vi "ReadForceSensor.vi"() -> ()   [LabVIEW 2011]
uses:
  sensor_list.ctl
  statesReadForceSensor.ctl
  QueueCtl.ctl
  <vilib>/DAQmx/read.llb/DAQmx Read (Analog DBL 1Chan 1Samp).vi
  <vilib>/DAQmx/create/channels.llb/DAQmx Create Channel (AI-Voltage-Basic).vi
  <vilib>/DAQmx/miscellaneous.llb/DAQmx Fill In Error Info.vi
  <vilib>/Utility/file.llb/Write To Spreadsheet File (DBL).vi
panel:
  in  "channels":tag
  in  "Previous":bool
  in  "Bumper":T1(ring)
  in  "Number of observations":i32=5
  in  "weight sequence (g)":dbl[](array[numeric])=[0.0, 50.0, 100.0, 200.0, 426.6, 1000.0, 1870.0, 2820.0, 3700.0, 5559.0, 6559.0, 7419.0, 9239.0]
  in  "Apparatus wt (g)":dbl=183.5
  in  "Unit number":string
  in  "Sensor model":T2=enum."interlink-FSR"
  out "standard error":string
  out "standard output":string
  in  "play python":bool
  in  "Data (CSV) path":path
  out "display":string="Remove all weights,\npull up the rod-setup and \npress \"NEXT\""
  in  "Next Button":bool
  out "Value (mV)":dbl
  out "Place weight (g)":dbl
  out "error out":errorcluster
  # "FORCE SENSOR - DEAD WEIGHT TEST"
  # "Settings:"
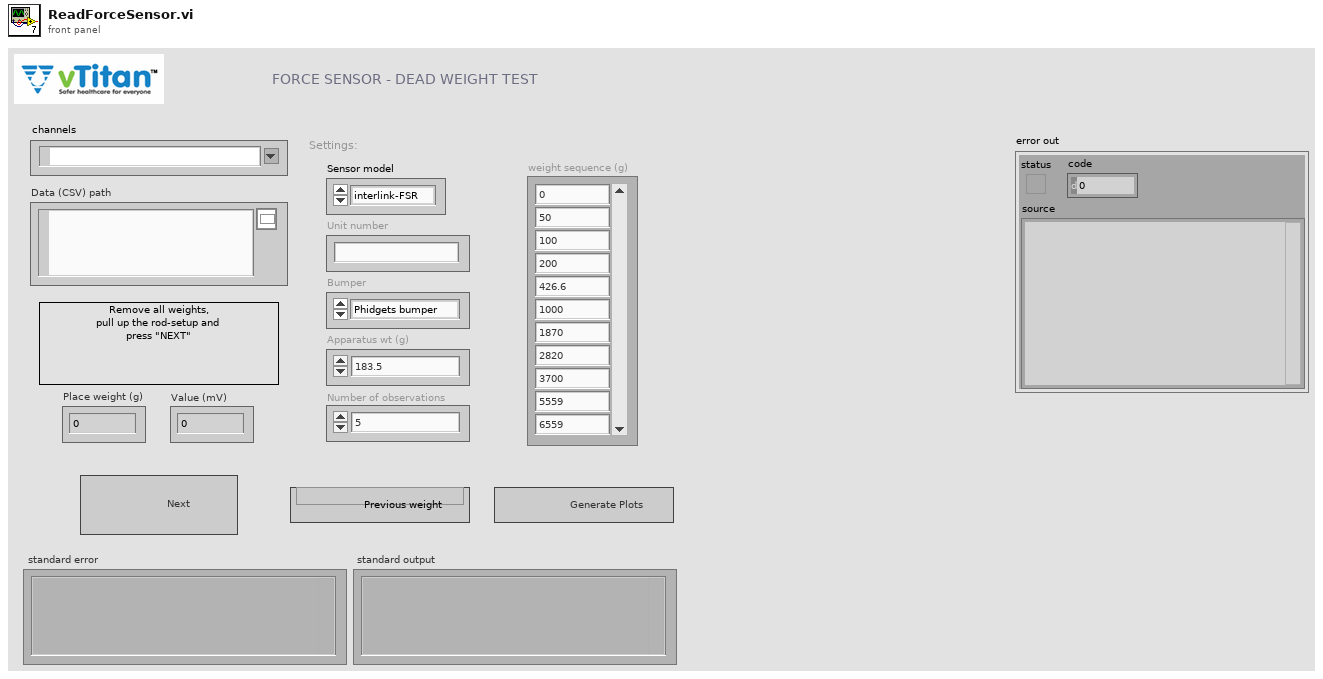
[diagram p1: front panel]
types:
  T1 = enum16{"Phidgets bumper", "Plastic bumper", "neoprene rubber"}
  T2 = typedef "sensor_list.ctl" = enum16{"ESS301", "FSG005WNPB", "FSG010WNPB", "FSG015WNPB", "FSS010WNGT", "FSS015WNGT", "A201", "interlink-FSR", "sensitronics-FSR", "NPI-12"}
  T3 = typedef "QueueCtl.ctl" = enum16{"Create", "Enqueue-N", "Dequeue - 1 ", "Enstack - N", "Flush", "Release"}
  T4 = cluster{"reading":dbl, "nul_offset":dbl, "device_ref":refnum<k21>, "weights":i32[], "data":dbl[][], "excel_path":path, "count":i32, "num_read":i32, "next":bool, "state_meas":enum16{"to_read_null", "to_read_value"}, "script_relpath":string}
  T5 = typedef "statesReadForceSensor.ctl" = enum16{"initialize", "poll", "find null offset", "measure value", "write to file", "remeasure weight", "display", "run python scripts", "exit"}
  T6 = enum16{"ESS301", "FSG005WNPB", "FSG010WNPB", "FSG015WNPB", "FSS010WNGT", "FSS015WNGT", "A201", "interlink-FSR", "sensitronics-FSR", "NPI-12"}
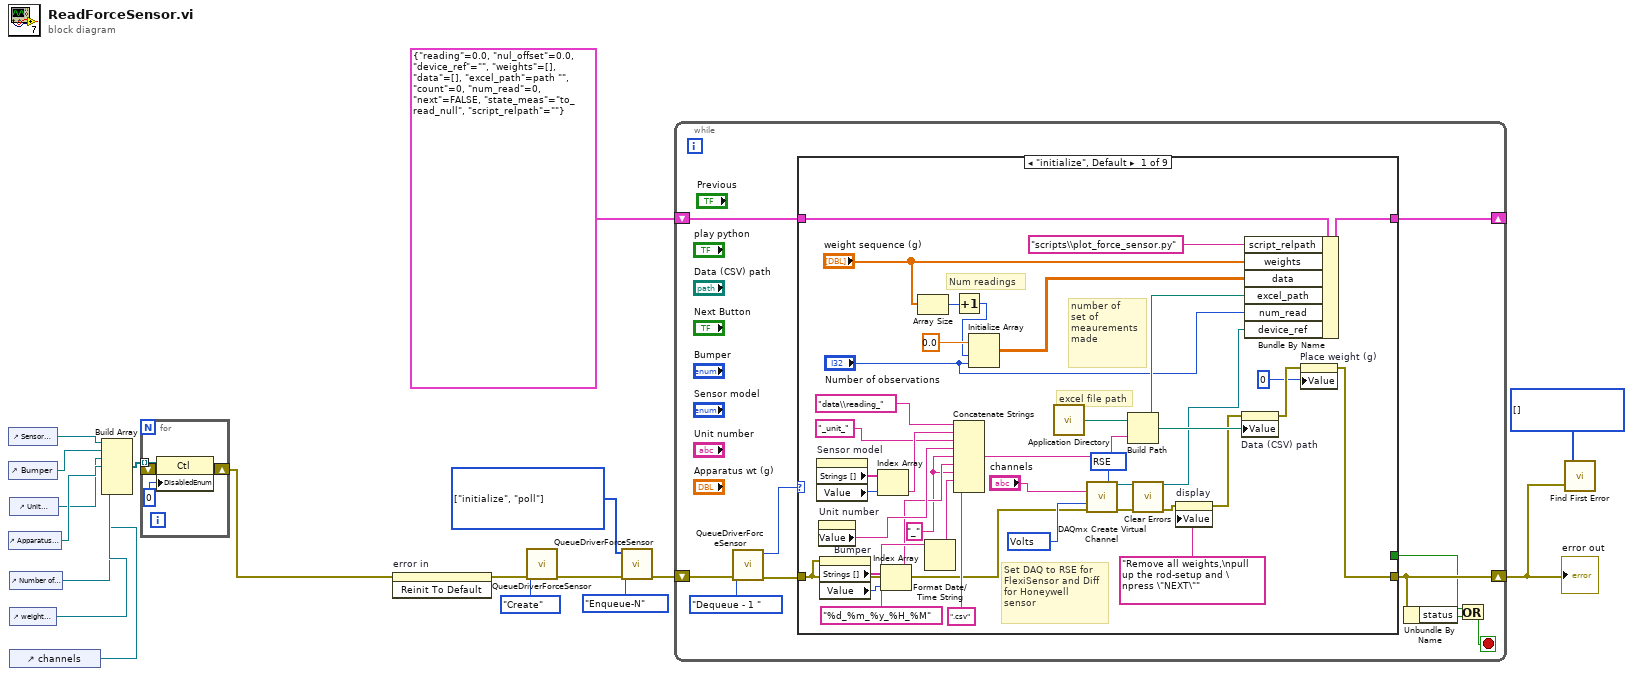
[diagram p0: block diagram]
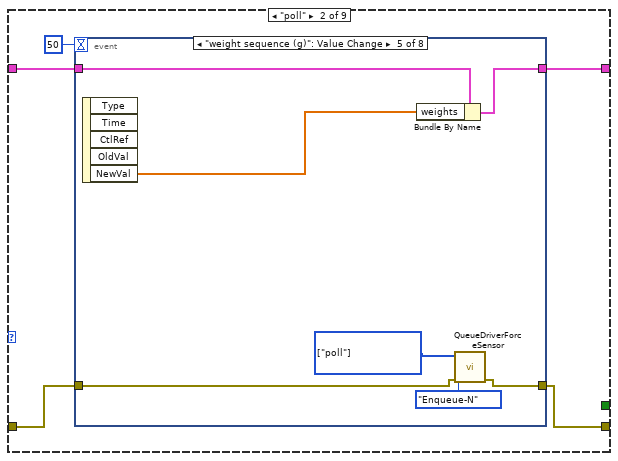
[diagram p2: hidden frame]
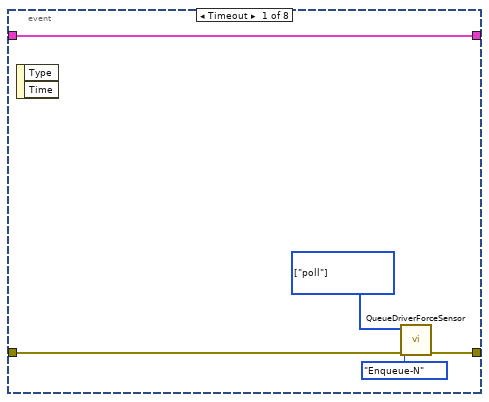
[diagram p3: hidden frame]
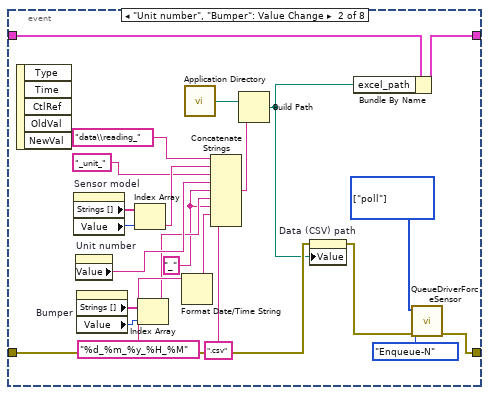
[diagram p4: hidden frame]
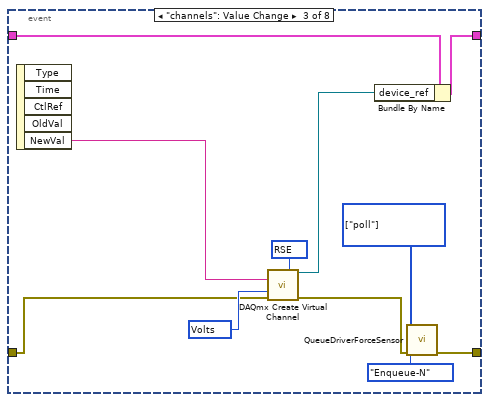
[diagram p5: hidden frame]
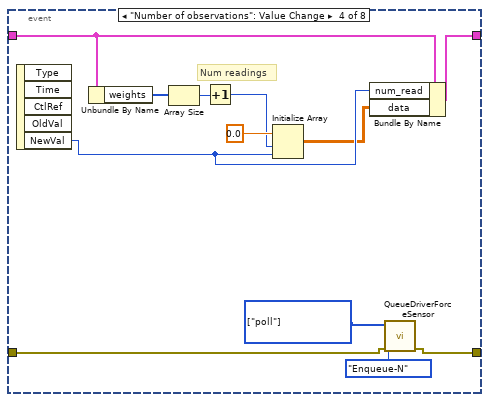
[diagram p6: hidden frame]
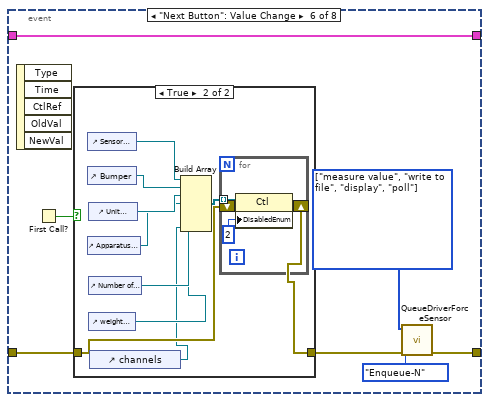
[diagram p7: hidden frame]
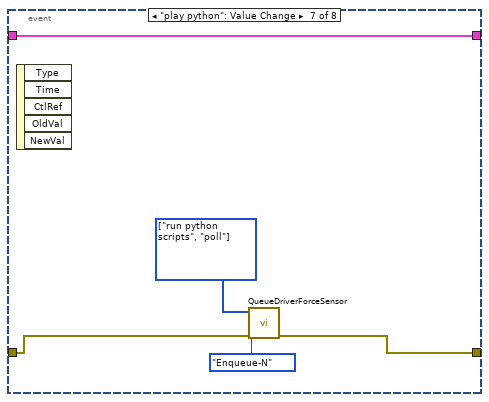
[diagram p9: hidden frame]
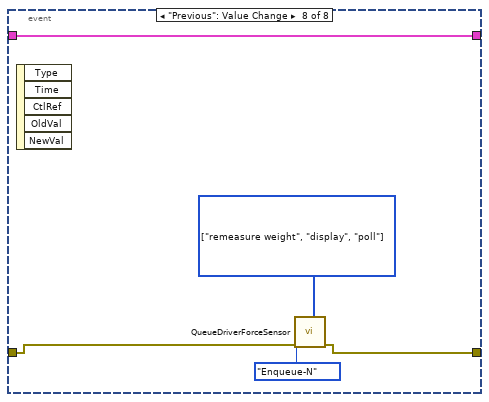
[diagram p10: hidden frame]
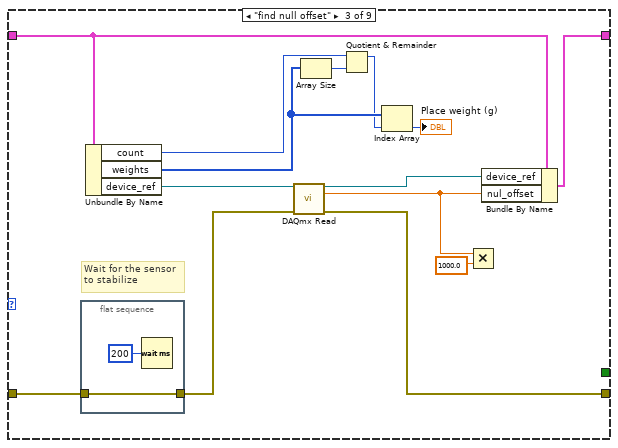
[diagram p11: hidden frame]
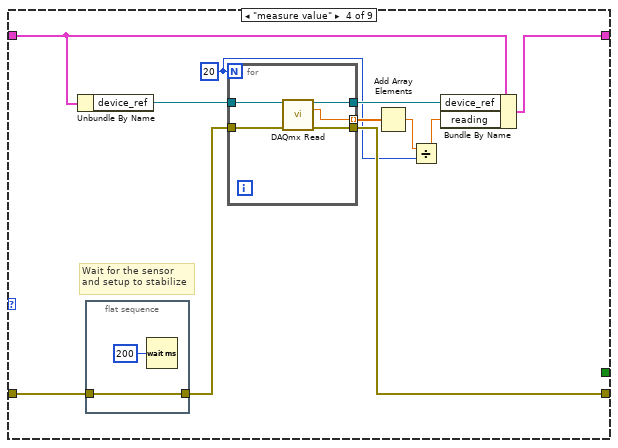
[diagram p12: hidden frame]
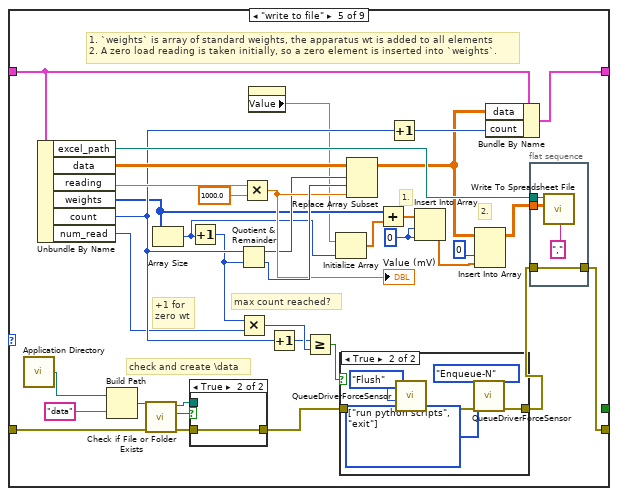
[diagram p13: hidden frame]
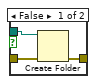
[diagram p15: hidden frame]
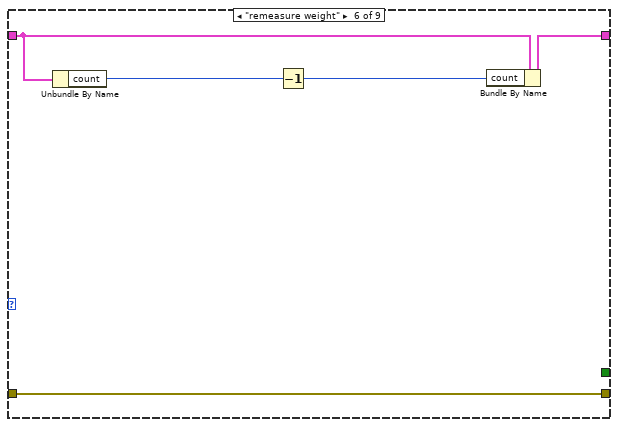
[diagram p16: hidden frame]
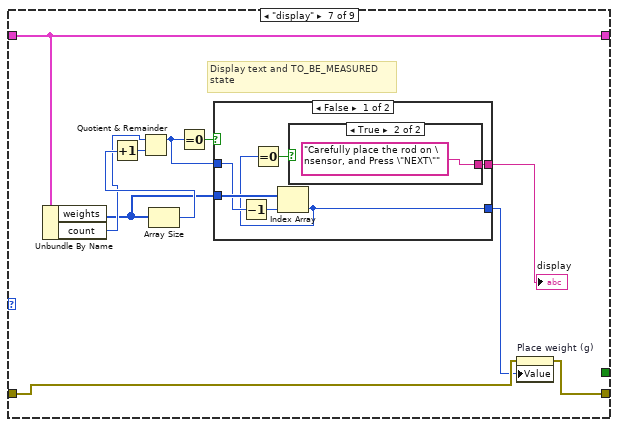
[diagram p17: hidden frame]
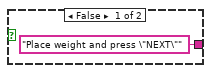
[diagram p18: hidden frame]
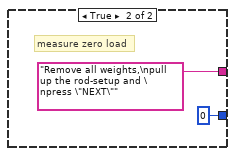
[diagram p19: hidden frame]
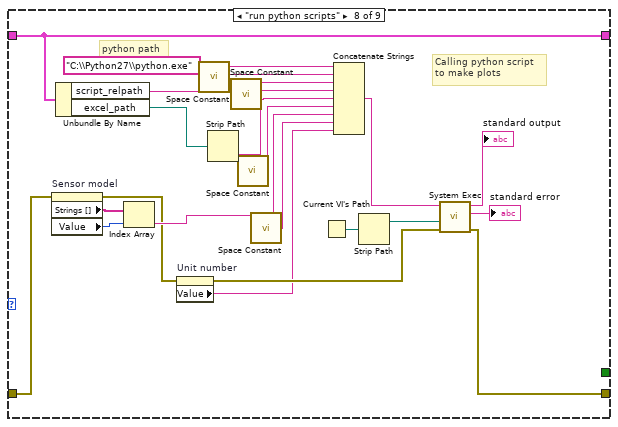
[diagram p20: hidden frame]
diagram:
  w11 = T5[] [enum."initialize", enum."poll"] items=["initialize", "poll", "find null offset", "measure value", "write to file", "remeasure weight", "display", "run python scripts", "exit"]
  n1 = control-ref of="Sensor model"() -> (w3:refnum<vi>)
  n2 = control-ref of="Bumper"() -> (w4:refnum<vi>)
  n3 = control-ref of="Apparatus wt (g)"() -> (w6:refnum<vi>)
  n4 = control-ref of="Unit number"() -> (w5:refnum<vi>)
  n5 = control-ref of="Number of observations"() -> (w7:refnum<vi>)
  n6 = control-ref of="weight sequence (g)"() -> (w8:refnum<vi>)
  n7 = control-ref of="channels"() -> (w1:refnum<vi>)
  n8 = Build Array(w3, w4, w5, w6, w7, w8, w1) -> (w9:refnum<vi>[])
  n9 = for {
    tunnel: w9 -> [w22] mode=indexing
    shift-right: [w19] -> w2
    shift-left: _ -> [w20]
    n10 = property class="Ctl"(reference=w22, error in=w20, "DisabledEnum"=0) -> (error out=w19:errorcluster)  [unwired: 1 out]
  }
  n11 = invoke on="error in" class="Clust (strict)" method="Reinit To Default"(error in=w2) -> (error out=w10:errorcluster)  [unwired: 2 in, 2 out]
  n12 = call "QueueDriverForceSensor.vi"("error in"=w10, "Enum"=QueueCtl."Create" ("Operation")) -> ("error in 2"=w14:errorcluster)  [unwired: 7 in, 2 out]
  n13 = call "QueueDriverForceSensor.vi"("error in"=w14, "Enum"=QueueCtl."Enqueue-N" ("Operation"), "Array"=w11) -> ("error in 2"=w12:errorcluster)  [unwired: 6 in, 2 out]
  n14 = while {
    shift-right: [w31] -> _
    shift-left: T4 {"reading"=0.0, "nul_offset"=0.0, "device_ref"="", "weights"=[], "data"=[], "excel_path"=path "", "count"=0, "num_read"=0, "next"=FALSE, "state_meas"=enum."to_read_null", "script_relpath"=""} -> [w32]
    shift-right: [w26] -> w17
    shift-left: w12 -> [w30]
    stop <- w25 stop-if-true
    n15 = call "QueueDriverForceSensor.vi"("error in"=w30, "Enum"=QueueCtl."Dequeue - 1 " ("Operation")) -> ("error in 2"=w29:errorcluster, "enum"=w27:T5)  [unwired: 7 in, 1 out]
    n16 = case shown="\"initialize\", Default" w27 {
      tunnel: w32 -> [w69 w72 w170 w189 w232 w254 w263 w295 w299]
      tunnel: [w68 w71 w178 w188 w231 w253 w263 w295 w299] -> w31
      tunnel: [w47 w70 w165 w187 w203 w250 w255 w276 w298] -> w26
      tunnel: w29 -> [w37 w73 w168 w186 w219 w250 w264 w284 w301]
      tunnel: [_ _ _ _ _ _ _ _ TRUE] -> w23
      frame "initialize", Default {
        w38 = 10083 items=["default"=-1, "RSE"=10083, "NRSE"=10078, "Differential"=10106, "Pseudodifferential"=12529] ("input terminal configuration")
        w39 = 10348 items=["Volts"=10348, "From Custom Scale"=10065] ("units")
        w41 = "_" ("string")
        # "Set DAQ to RSE for\nFlexiSensor and Diff\nfor Honeywell\nsensor"
        # "number of\nset of meaurements made"
        # "excel file path"
        # "Num readings"
        n17 = property on="Sensor model" class="Enum (strict)"() -> ("Strings []"=w50:string[], "Value"=w51:T6)  [unwired: 2 in, 2 out]
        n18 = property on="Unit number" class="Str"() -> ("Value"=w46:string)  [unwired: 2 in, 2 out]
        n19 = property on="Bumper" class="Enum (strict)"(error in=w37) -> ("Strings []"=w45:string[], "Value"=w44:T1)  [unwired: 1 in, 2 out]
        n20 = Index Array(array=w50, index=w51) -> (element=w49:string)
        n21 = Index Array(array=w45, index=w44) -> (element=w43:string)
        n22 = Array Size(array="weight sequence (g)") -> (size(s)=w55:i32)
        n23 = Format Date/Time String(time format string (%c)="%d_%m_%y_%H_%M") -> (date/time string=w42:string)  [unwired: 2 in]
        n24 = Increment(x=w55) -> (x+1=w54:i32)
        n25 = Concatenate Strings("data\\reading_" ("name or relative path"), w49, "_unit_" ("string"), w46, w41, w43, w41, w42, ".csv" ("name or relative path")) -> (w62:string)
        n26 = Initialize Array(0.0, w54, "Number of observations") -> (w66:dbl[][])
        n27 = call <vilib>:"Application Directory.vi"() -> ("Application Directory"=w40:path)
        n28 = call-poly <vilib>:"DAQmx Create Virtual Channel.vi"("input terminal configuration"=w38, "physical channels"="channels", "units"=w39, "error in"=w37) -> ("task out"=w35:refnum<k21>, "error out"=w34:errorcluster)  [unwired: 10 in]
        n29 = Build Path(base path=w40, name or relative path=w62) -> (appended path=w65:path)
        n30 = call <vilib>:"Clear Errors.vi"("error in (no error)"=w34) -> ("error out"=w33:errorcluster)  [unwired: 6 in]
        n31 = property on="display" class="Str"(error in=w33, "Value"="Remove all weights,\npull up the rod-setup and \npress \"NEXT\"" ("display")) -> (error out=w60:errorcluster)  [unwired: 1 in, 1 out]
        n32 = property on="Data (CSV) path" class="Path"(error in=w60, "Value"=w65) -> (error out=w57:errorcluster)  [unwired: 1 in, 1 out]
        n33 = Bundle By Name(cluster=w69, "script_relpath"="scripts\\plot_force_sensor.py" ("python_script_name"), "weights"="weight sequence (g)", "data"=w66, "excel_path"=w65, "num_read"="Number of observations", "device_ref"=w35) -> (w68:T4)
        n34 = property on="Place weight (g)" class="DigNum (strict)"(error in=w57, "Value"=0 ("dimension size")) -> (error out=w47:errorcluster)  [unwired: 1 in, 1 out]
      }
      frame "poll" {
        n35 = event shown="[4] \"weight sequence (g)\": Value Change" {
          selector: _ -> [_ _ _ _ _ _ _ _]
          dyn-events: _ -> [_ _ _ _ _ _ _ _]
          timeout: 50 -> [_ _ _ _ _ _ _ _]
          tunnel: w73 -> [w78 w87 w112 w115 w126 w134 w158 w162]
          tunnel: [w77 w80 w104 w116 w127 w136 w156 w161] -> w70
          tunnel: w72 -> [w79 w89 w109 w121 w132 w139 w159 w160]
          tunnel: [w79 w88 w108 w120 w131 w139 w159 w160] -> w71
          event Timeout {
            w75 = T5[] [enum."poll"] items=["initialize", "poll", "find null offset", "measure value", "write to file", "remeasure weight", "display", "run python scripts", "exit"]
            n36 = event-data() -> ()  [unwired: 1 in, 2 out]
            n37 = call "QueueDriverForceSensor.vi"("error in"=w78, "Enum"=QueueCtl."Enqueue-N" ("Operation"), "Array"=w75) -> ("error in 2"=w77:errorcluster)  [unwired: 6 in, 2 out]
          }
          event "Unit number", "Bumper": Value Change {
            w82 = T5[] [enum."poll"] items=["initialize", "poll", "find null offset", "measure value", "write to file", "remeasure weight", "display", "run python scripts", "exit"]
            w90 = "_" ("string")
            n38 = event-data() -> ()  [unwired: 1 in, 5 out]
            n39 = property on="Sensor model" class="Enum (strict)"() -> ("Strings []"=w98:string[], "Value"=w99:T6)  [unwired: 2 in, 2 out]
            n40 = property on="Unit number" class="Str"() -> ("Value"=w95:string)  [unwired: 2 in, 2 out]
            n41 = property on="Bumper" class="Enum (strict)"() -> ("Strings []"=w94:string[], "Value"=w93:T1)  [unwired: 2 in, 2 out]
            n42 = Index Array(array=w98, index=w99) -> (element=w97:string)
            n43 = Index Array(array=w94, index=w93) -> (element=w92:string)
            n44 = Format Date/Time String(time format string (%c)="%d_%m_%y_%H_%M") -> (date/time string=w91:string)  [unwired: 2 in]
            n45 = call <vilib>:"Application Directory.vi"() -> ("Application Directory"=w84:path)
            n46 = Concatenate Strings("data\\reading_" ("name or relative path"), w97, "_unit_" ("string"), w95, w90, w92, w90, w91, ".csv" ("name or relative path")) -> (w86:string)
            n47 = Build Path(base path=w84, name or relative path=w86) -> (appended path=w85:path)
            n48 = property on="Data (CSV) path" class="Path"(error in=w87, "Value"=w85) -> (error out=w81:errorcluster)  [unwired: 1 in, 1 out]
            n49 = Bundle By Name(cluster=w89, "excel_path"=w85) -> (w88:T4)
            n50 = call "QueueDriverForceSensor.vi"("error in"=w81, "Enum"=QueueCtl."Enqueue-N" ("Operation"), "Array"=w82) -> ("error in 2"=w80:errorcluster)  [unwired: 6 in, 2 out]
          }
          event "channels": Value Change {
            w105 = T5[] [enum."poll"] items=["initialize", "poll", "find null offset", "measure value", "write to file", "remeasure weight", "display", "run python scripts", "exit"]
            w111 = 10083 items=["default"=-1, "RSE"=10083, "NRSE"=10078, "Differential"=10106, "Pseudodifferential"=12529] ("input terminal configuration")
            w113 = 10348 items=["Volts"=10348, "From Custom Scale"=10065] ("units")
            n51 = event-data() -> ("NewVal"=w110:tag)  [unwired: 1 in, 4 out]
            n52 = call-poly <vilib>:"DAQmx Create Virtual Channel.vi"("input terminal configuration"=w111, "physical channels"=w110, "units"=w113, "error in"=w112) -> ("task out"=w107:refnum<k21>, "error out"=w103:errorcluster)  [unwired: 10 in]
            n53 = Bundle By Name(cluster=w109, "device_ref"=w107) -> (w108:T4)
            n54 = call "QueueDriverForceSensor.vi"("error in"=w103, "Enum"=QueueCtl."Enqueue-N" ("Operation"), "Array"=w105) -> ("error in 2"=w104:errorcluster)  [unwired: 6 in, 2 out]
          }
          event "Number of observations": Value Change {
            w114 = T5[] [enum."poll"] items=["initialize", "poll", "find null offset", "measure value", "write to file", "remeasure weight", "display", "run python scripts", "exit"] ("Array")
            # "Num readings"
            n55 = event-data() -> ("NewVal"=w119:i32)  [unwired: 1 in, 4 out]
            n56 = Unbundle By Name(w121) -> ("weights"=w122:i32[])
            n57 = Array Size(array=w122) -> (size(s)=w124:i32)
            n58 = Increment(x=w124) -> (x+1=w123:i32)
            n59 = Initialize Array(0.0, w123, w119) -> (w118:dbl[][])
            n60 = Bundle By Name(cluster=w121, "num_read"=w119, "data"=w118) -> (w120:T4)
            n61 = call "QueueDriverForceSensor.vi"("error in"=w115, "Enum"=QueueCtl."Enqueue-N" ("Operation"), "Array"=w114) -> ("error in 2"=w116:errorcluster)  [unwired: 6 in, 2 out]
          }
          event "weight sequence (g)": Value Change {
            w128 = T5[] [enum."poll"] items=["initialize", "poll", "find null offset", "measure value", "write to file", "remeasure weight", "display", "run python scripts", "exit"] ("Array")
            n62 = event-data() -> ("NewVal"=w130:dbl[])  [unwired: 1 in, 4 out]
            n63 = Bundle By Name(cluster=w132, "weights"=w130) -> (w131:T4)
            n64 = call "QueueDriverForceSensor.vi"("error in"=w126, "Enum"=QueueCtl."Enqueue-N" ("Operation"), "Array"=w128) -> ("error in 2"=w127:errorcluster)  [unwired: 6 in, 2 out]
          }
          event "Next Button": Value Change {
            w137 = T5[] [enum."measure value", enum."write to file", enum."display", enum."poll"] items=["initialize", "poll", "find null offset", "measure value", "write to file", "remeasure weight", "display", "run python scripts", "exit"]
            n65 = event-data() -> ()  [unwired: 1 in, 5 out]
            n66 = First Call?() -> (First Call?: T/F=w135:bool)
            n67 = case shown="True" w135 {
              tunnel: [w140 w142] -> w133
              tunnel: w134 -> [w140 w143]
              frame False {
              }
              frame True {
                n68 = control-ref of="Sensor model"() -> (w150:refnum<vi>)
                n69 = control-ref of="Bumper"() -> (w149:refnum<vi>)
                n70 = control-ref of="Apparatus wt (g)"() -> (w147:refnum<vi>)
                n71 = control-ref of="Unit number"() -> (w148:refnum<vi>)
                n72 = control-ref of="Number of observations"() -> (w146:refnum<vi>)
                n73 = control-ref of="weight sequence (g)"() -> (w145:refnum<vi>)
                n74 = control-ref of="channels"() -> (w141:refnum<vi>)
                n75 = Build Array(w150, w149, w148, w147, w146, w145, w141) -> (w144:refnum<vi>[])
                n76 = for {
                  tunnel: w144 -> [w154] mode=indexing
                  shift-right: [w151] -> w142
                  shift-left: w143 -> [w152]
                  n77 = property class="Ctl"(reference=w154, error in=w152, "DisabledEnum"=2) -> (error out=w151:errorcluster)  [unwired: 1 out]
                }
              }
            }
            n78 = call "QueueDriverForceSensor.vi"("error in"=w133, "Enum"=QueueCtl."Enqueue-N" ("Operation"), "Array"=w137) -> ("error in 2"=w136:errorcluster)  [unwired: 6 in, 2 out]
          }
          event "play python": Value Change {
            w155 = T5[] [enum."run python scripts", enum."poll"] items=["initialize", "poll", "find null offset", "measure value", "write to file", "remeasure weight", "display", "run python scripts", "exit"]
            n79 = event-data() -> ()  [unwired: 1 in, 5 out]
            n80 = call "QueueDriverForceSensor.vi"("error in"=w158, "Enum"=QueueCtl."Enqueue-N" ("Operation"), "Array"=w155) -> ("error in 2"=w156:errorcluster)  [unwired: 6 in, 2 out]
          }
          event "Previous": Value Change {
            w163 = T5[] [enum."remeasure weight", enum."display", enum."poll"] items=["initialize", "poll", "find null offset", "measure value", "write to file", "remeasure weight", "display", "run python scripts", "exit"]
            n81 = event-data() -> ()  [unwired: 1 in, 5 out]
            n82 = call "QueueDriverForceSensor.vi"("error in"=w162, "Enum"=QueueCtl."Enqueue-N" ("Operation"), "Array"=w163) -> ("error in 2"=w161:errorcluster)  [unwired: 6 in, 2 out]
          }
        }
      }
      frame "find null offset" {
        # "Wait for the sensor\nto stabilize"
        n83 = flat-sequence {
          tunnel: w168 -> [w180]
          tunnel: [w180] -> w169
          frame #0 {
            n84 = Wait (ms)(milliseconds to wait=u32 200) -> ()  [unwired: 1 out]
          }
        }
        n85 = Unbundle By Name(w170) -> ("count"=w175:i32, "weights"=w172:i32[], "device_ref"=w177:refnum<k21>)
        n86 = call-poly <vilib>:"DAQmx Read.vi"("task/channels in"=w177, "error in"=w169) -> ("task out"=w176:refnum<k21>, "data"=w166:dbl, "error out"=w165:errorcluster)  [unwired: 11 in]
        n87 = Array Size(array=w172) -> (size(s)=w174:i32)
        n88 = Quotient & Remainder(x=w175, y=w174) -> (x-y*floor(x/y)=w171:i32)  [unwired: 1 out]
        n89 = Index Array(array=w172, index=w171) -> (element=→"Place weight (g)":i32)
        n90 = Multiply(x=w166, y=1000.0) -> ()  [unwired: 1 out]
        n91 = Bundle By Name(cluster=w170, "device_ref"=w176, "nul_offset"=w166) -> (w178:T4)
      }
      frame "measure value" {
        w182 = 20
        # "Wait for the sensor\nand setup to stabilize"
        n92 = Unbundle By Name(w189) -> ("device_ref"=w190:refnum<k21>)
        n93 = flat-sequence {
          tunnel: w186 -> [w198]
          tunnel: [w198] -> w185
          frame #0 {
            n94 = Wait (ms)(milliseconds to wait=u32 200) -> ()  [unwired: 1 out]
          }
        }
        n95 = for {
          N: w182 -> [_]
          tunnel: [w196] -> w191
          tunnel: w190 -> [w195]
          tunnel: [w194] -> w187
          tunnel: w185 -> [w193]
          tunnel: [w192] -> w184 mode=indexing
          n96 = call-poly <vilib>:"DAQmx Read.vi"("task/channels in"=w195, "error in"=w193) -> ("task out"=w196:refnum<k21>, "data"=w192:dbl, "error out"=w194:errorcluster)  [unwired: 11 in]
        }
        n97 = Add Array Elements(numeric array=w184) -> (sum=w183:dbl)
        n98 = Divide(x=w183, y=w182) -> (x/y=w181:dbl)
        n99 = Bundle By Name(cluster=w189, "device_ref"=w191, "reading"=w181) -> (w188:T4)
      }
      frame "write to file" {
        w207 = 0 ("index")
        # "1. `weights` is array of standard weights, the apparatus wt is added to all elements\n2. A zero load reading is taken initially, so a zero element is inserted into `weights`."
        # "2."
        # "1."
        # "+1 for \nzero wt"
        # "check and create \\data"
        # "max count reached?"
        n100 = call <vilib>:"Application Directory.vi"() -> ("Application Directory"=w199:path)
        n101 = Unbundle By Name(w232) -> ("excel_path"=w233:path, "data"=w234:dbl[][], "reading"=w228:dbl, "weights"=w212:i32[], "count"=w222:i32, "num_read"=w221:i32)
        n102 = Build Path(base path=w199, name or relative path="data") -> (appended path=w215:path)
        n103 = call <vilib>:"Check if File or Folder Exists.vi"("error in (no error)"=w219, "path"=w215) -> ("error out"=w218:errorcluster, "file or folder exists?"=w217:bool, "dup path"=w216:path)  [unwired: 7 in]
        n104 = Array Size(array=w212) -> (size(s)=w210:i32)
        n105 = Increment(x=w210) -> (x+1=w213:i32)
        n106 = case shown="True" w217 {
          tunnel: w218 -> [w248 w249]
          tunnel: [w247 w249] -> w202
          tunnel: w216 -> [w246 _]
          frame False {
            n107 = Create Folder(path (use dialog)=w246, error in=w248) -> (error out=w247:errorcluster)  [unwired: 1 in, 2 out]
          }
          frame True {
          }
        }
        n108 = Quotient & Remainder(x=w222, y=w213) -> (x-y*floor(x/y)=w225:i32, floor(x/y)=w229:i32)
        n109 = Multiply(x=w213, y=w221) -> (x*y=w224:i32)
        n110 = Multiply(x=w228, y=1000.0) -> (x*y=w226:dbl)
        "Value (mV)" <- w226
        n111 = property on="Apparatus wt (g)" class="DigNum (strict)"() -> ("Value"=w211:dbl)  [unwired: 2 in, 2 out]
        n112 = Increment(x=w222) -> (x+1=w223:i32)
        n113 = Greater Or Equal?(x=w223, y=w224) -> (x >= y?=w201:bool)
        n114 = Initialize Array(w211, w210) -> (w209:dbl[])
        n115 = case shown="True" w201 {
          tunnel: w202 -> [w235 w241]
          tunnel: [w235 w237] -> w200
          frame False {
          }
          frame True {
            w236 = T5[] [enum."run python scripts", enum."exit"] items=["initialize", "poll", "find null offset", "measure value", "write to file", "remeasure weight", "display", "run python scripts", "exit"] ("t")
            n116 = call "QueueDriverForceSensor.vi"("error in"=w241, "Enum"=QueueCtl."Flush") -> ("error in 2"=w238:errorcluster)  [unwired: 7 in, 2 out]
            n117 = call "QueueDriverForceSensor.vi"("error in"=w238, "Enum"=QueueCtl."Enqueue-N" ("Operation"), "Array"=w236) -> ("error in 2"=w237:errorcluster)  [unwired: 6 in, 2 out]
          }
        }
        n118 = Replace Array Subset(array=w234, new element=w226, index (row)=w225, index (col)=w229) -> (w204:dbl[][])
        n119 = Add(x=w212, y=w209) -> (x+y=w208:dbl[])
        n120 = Increment(x=w222) -> (x+1=w230:i32)
        n121 = Insert Into Array(array=w208, index=w207, new element=w207) -> (w206:dbl[])
        n122 = Insert Into Array(array=w204, index (col)=0 ("disabled index (col)"), new element=w206) -> (w205:dbl[][])  [unwired: 1 in]
        n123 = Bundle By Name(cluster=w232, "data"=w204, "count"=w230) -> (w231:T4)
        n124 = flat-sequence {
          tunnel: w233 -> [w245]
          tunnel: w205 -> [w243]
          tunnel: w200 -> [w242]
          tunnel: [w242] -> w203
          frame #0 {
            n125 = call-poly <vilib>:"Write To Spreadsheet File.vi"("delimiter (\\t)"="," ("delimiter (\\t)"), "2D data"=w243, "file path (dialog if empty)"=w245) -> ()  [unwired: 5 in, 1 out]
          }
        }
      }
      frame "remeasure weight" {
        n126 = Unbundle By Name(w254) -> ("count"=w252:i32)
        n127 = Decrement(x=w252) -> (x-1=w251:i32)
        n128 = Bundle By Name(cluster=w254, "count"=w251) -> (w253:T4)
      }
      frame "display" {
        # "Display text and TO_BE_MEASURED\nstate"
        n129 = Unbundle By Name(w263) -> ("weights"=w257:i32[], "count"=w259:i32)
        n130 = Array Size(array=w257) -> (size(s)=w261:i32)
        n131 = Increment(x=w261) -> (x+1=w260:i32)
        n132 = Quotient & Remainder(x=w259, y=w260) -> (x-y*floor(x/y)=w258:i32)  [unwired: 1 out]
        n133 = Equal To 0?(x=w258) -> (x = 0?=w262:bool)
        n134 = case shown="False" w262 {
          tunnel: [w271 "Remove all weights,\npull up the rod-setup and \npress \"NEXT\"" ("display")] -> w265
          tunnel: w258 -> [w269 _]
          tunnel: w257 -> [w270 _]
          tunnel: [w267 0 ("index")] -> w256
          frame False {
            n135 = Decrement(x=w269) -> (x-1=w268:i32)
            n136 = Index Array(array=w270, index=w268) -> (element=w267:i32)
            n137 = Equal To 0?(x=w267) -> (x = 0?=w266:bool)
            n138 = case shown="True" w266 {
              tunnel: ["Place weight and press \"NEXT\"" ("display") "Carefully place the rod on \nsensor, and Press \"NEXT\"" ("display")] -> w271
              frame False {
              }
              frame True {
              }
            }
          }
          frame True {
            # "measure zero load"
          }
        }
        "display" <- w265
        n139 = property on="Place weight (g)" class="DigNum (strict)"(error in=w264, "Value"=w256) -> (error out=w255:errorcluster)  [unwired: 1 in, 1 out]
      }
      frame "run python scripts" {
        # "python path"
        # "Calling python script\nto make plots"
        n140 = property on="Sensor model" class="Enum (strict)"(error in=w284) -> (error out=w280:errorcluster, "Strings []"=w283:string[], "Value"=w282:T6)  [unwired: 1 in, 1 out]
        n141 = Unbundle By Name(w295) -> ("script_relpath"=w292:string, "excel_path"=w287:path)
        n142 = Index Array(array=w283, index=w282) -> (element=w281:string)
        n143 = property on="Unit number" class="Str"(error in=w280) -> (error out=w279:errorcluster, "Value"=w277:string)  [unwired: 1 in, 1 out]
        n144 = call <vilib>:"Space Constant.vi"() -> ("String"=w293:string)
        n145 = Strip Path(path=w287) -> (name=w286:string)  [unwired: 1 out]
        n146 = call <vilib>:"Space Constant.vi"() -> ("String"=w291:string)
        n147 = call <vilib>:"Space Constant.vi"() -> ("String"=w285:string)
        n148 = call <vilib>:"Space Constant.vi"() -> ("String"=w278:string)
        n149 = Current VI's Path() -> (path=w297:path)
        n150 = Concatenate Strings("C:\\Python27\\python.exe" ("command line"), w293, w292, w291, w286, w285, w281, w278, w277) -> (w290:string)
        n151 = Strip Path(path=w297) -> (stripped path=w296:path)  [unwired: 1 out]
        n152 = call <vilib>:"System Exec.vi"("error in (no error)"=w279, "working directory"=w296, "command line"=w290) -> ("error out"=w276:errorcluster, "standard error"=→"standard error":string, "standard output"=→"standard output":string)  [unwired: 5 in, 1 out]
      }
      frame "exit" {
        n153 = Unbundle By Name(w299) -> ("device_ref"=w302:refnum<k21>)
        n154 = call <vilib>:"DAQmx Clear Task.vi"("task in"=w302, "error in"=w301) -> ("error out"=w298:errorcluster)  [unwired: 13 in]
      }
    }
    n155 = Unbundle By Name(w26) -> ("status"=w24:bool)
    n156 = Or(x=w23, y=w24) -> (x .or. y?=w25:bool)
  }
  "error out" <- w17
  n157 = call <vilib>:"Find First Error.vi"("error in (no error)"=w17, "error codes"=i32[] []) -> ()  [unwired: 2 in, 2 out]
